vi "Alarms Test Bench.vi"() -> ()   [LabVIEW 2014]
uses:
  Controls/Alarms Data.ctl
  Controls/Modbus Status Interface Data MOD2.ctl
panel:
  in  "Clear Alarms In":bool=TRUE
  in  "MSI Data":T1 {"Converter Faults (30056)" format="%016b"; "Solar Faults (30057)" format="%016b"; "ES Rack 10 Alarms (30120)" format="%016b"; "ES Rack 9 Alarms (30119)" format="%016b"; "ES Rack 8 Alarms (30118)" format="%016b"; "ES Rack 7 Alarms (30117)" format="%016b"; "ES Rack 6 Alarms (30116)" format="%016b"; "ES Rack 5 Alarms (30115)" format="%016b"; "ES Rack 4 Alarms (30114)" format="%016b"; "ES Rack 3 Alarms (30113)" format="%016b"; "ES Rack 2 Alarms (30112)" format="%016b"; "ES Rack 1 Alarms (30111)" format="%016b"; "ES System Alarms (30055)" format="%016b"; "System Faults (30052)" format="%016b"; "ES Rack 10 Faults (30110)" format="%016b"; "Es Rack 9 Faults (30109)" format="%016b"; "ES Rack 8 Faults (30108)" format="%016b"; "ES Rack 7  Faults (30107)" format="%016b"; "ES Rack 6 Faults (30106)" format="%016b"; "ES Rack 5 Faults (30105)" format="%016b"; "ES Rack 4 Faults (30104)" format="%016b"; "ES Rack 3 Faults (30103)" format="%016b"; "ES Rack 2 Faults (30102)" format="%016b"; "ES Rack 1 Faults (30101)" format="%016b"; "ES System Faults (30054)" format="%016b"; "System Status (30051)" format="%016b"; "Controller Faults (30053)" format="%016b"}
  out "Alarms Data Out":T2
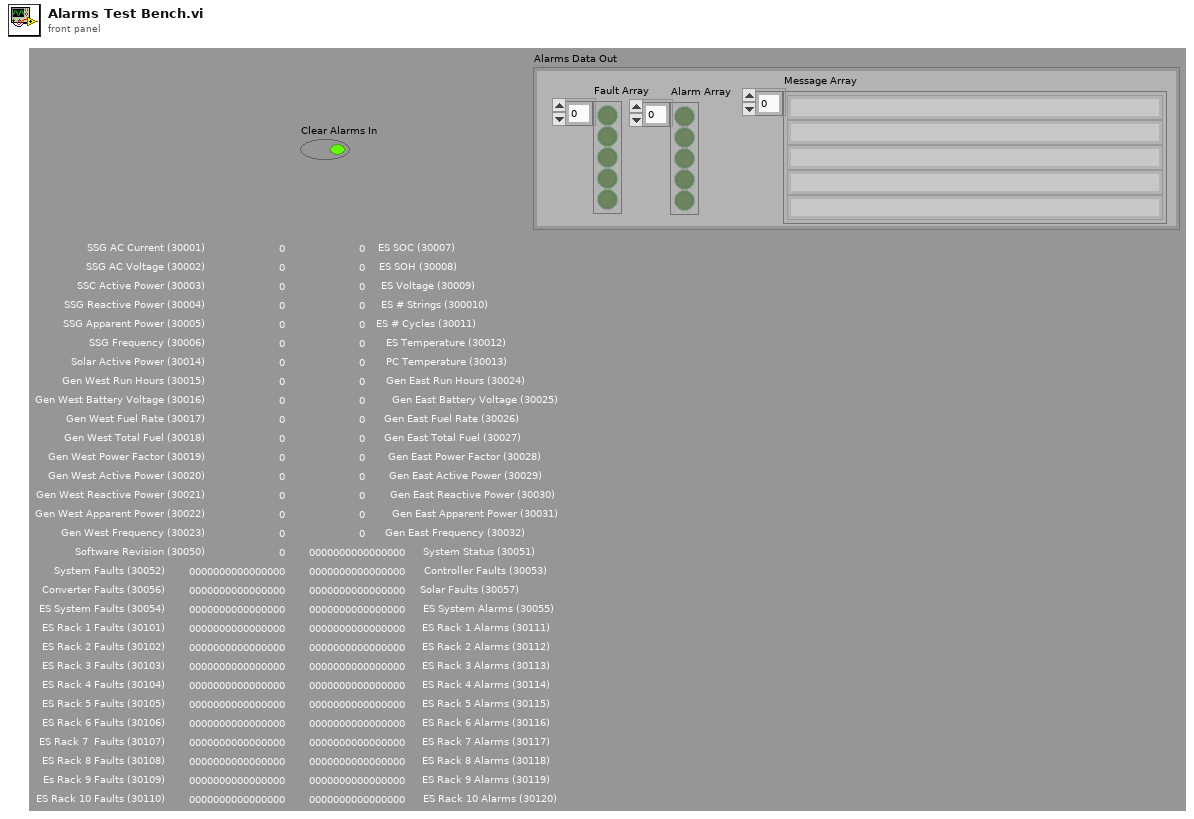
[diagram p1: front panel]
types:
  T1 = typedef "Modbus Status Interface Data MOD2.ctl" = cluster{"SSG AC Current (30001)":i16, "SSG AC Voltage (30002)":i16, "SSC Active Power (30003)":i16, "SSG Reactive Power (30004)":i16, "SSG Apparent Power (30005)":i16, "SSG Frequency (30006)":i16, "ES SOC (30007)":i16, "ES SOH (30008)":i16, "ES Voltage (30009)":i16, "ES # Strings (300010)":i16, "ES # Cycles (30011)":i16, "ES Temperature (30012)":i16, "PC Temperature (30013)":i16, "Solar Active Power (30014)":i16, "Gen West Run Hours (30015)":i16, "Gen West Battery Voltage (30016)":i16, "Gen West Fuel Rate (30017)":i16, "Gen West Total Fuel (30018)":i16, "Gen West Power Factor (30019)":i16, "Gen West Active Power (30020)":i16, "Gen West Reactive Power (30021)":i16, "Gen West Apparent Power (30022)":i16, "Gen West Frequency (30023)":i16, "Gen East Run Hours (30024)":i16, "Gen East Battery Voltage (30025) ":i16, "Gen East Fuel Rate (30026)":i16, "Gen East Total Fuel (30027)":i16, "Gen East Power Factor (30028)":i16, "Gen East Active Power (30029)":i16, "Gen East Reactive Power (30030)":i16, "Gen East Apparent Power (30031)":i16, "Gen East Frequency (30032)":i16, "Software Revision (30050)":i16, "Controller Faults (30053)":i16, "System Status (30051)":i16, "ES System Faults (30054)":i16, "ES Rack 1 Faults (30101)":i16, "ES Rack 2 Faults (30102)":i16, "ES Rack 3 Faults (30103)":i16, "ES Rack 4 Faults (30104)":i16, "ES Rack 5 Faults (30105)":i16, "ES Rack 6 Faults (30106)":i16, "ES Rack 7  Faults (30107)":i16, "ES Rack 8 Faults (30108)":i16, "Es Rack 9 Faults (30109)":i16, "ES Rack 10 Faults (30110)":i16, "System Faults (30052)":i16, "ES System Alarms (30055)":i16, "ES Rack 1 Alarms (30111)":i16, "ES Rack 2 Alarms (30112)":i16, "ES Rack 3 Alarms (30113)":i16, "ES Rack 4 Alarms (30114)":i16, "ES Rack 5 Alarms (30115)":i16, "ES Rack 6 Alarms (30116)":i16, "ES Rack 7 Alarms (30117)":i16, "ES Rack 8 Alarms (30118)":i16, "ES Rack 9 Alarms (30119)":i16, "ES Rack 10 Alarms (30120)":i16, "Solar Faults (30057)":i16, "Converter Faults (30056)":i16}
  T2 = typedef "Alarms Data.ctl" = cluster{"Message Array":string[], "Fault Array":bool[], "Alarm Array":bool[]}
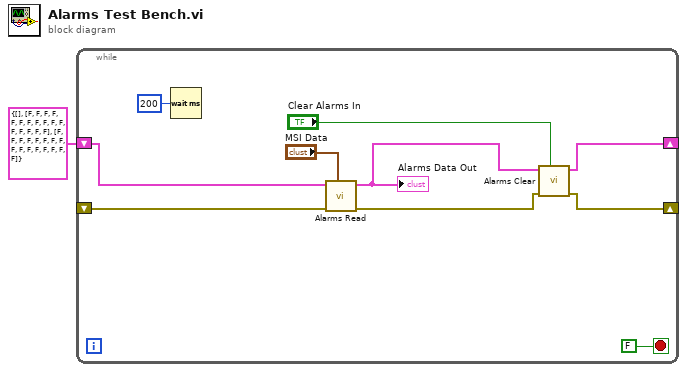
[diagram p0: block diagram]
diagram:
  n1 = while {
    shift-right: [w3] -> _
    shift-left: _ -> [w11]
    shift-right: [w5] -> _
    shift-left: T2 {"Message Array"=[], "Fault Array"=[FALSE, FALSE, FALSE, FALSE, FALSE, FALSE, FALSE, FALSE, FALSE, FALSE, FALSE, FALSE, FALSE, FALSE, FALSE, FALSE], "Alarm Array"=[FALSE, FALSE, FALSE, FALSE, FALSE, FALSE, FALSE, FALSE, FALSE, FALSE, FALSE, FALSE, FALSE, FALSE, FALSE, FALSE]} ("Alarms Data Out") -> [w7]
    stop <- FALSE stop-if-true
    n2 = Wait (ms)(milliseconds to wait=u32 200) -> ()  [unwired: 1 out]
    n3 = call "Alarms Read.vi"("MSI Data"="MSI Data", "Error In"=w11, "Alarms Data In"=w7) -> ("Error Out"=w4:errorcluster, "Alarms Data Out"=w6:T2)  [unwired: 7 in]
    "Alarms Data Out" <- w6
    n4 = call "Alarms Clear.vi"("Clear Alarms In"="Clear Alarms In", "Error In"=w4, "Alarms Data In"=w6) -> ("Error Out"=w3:errorcluster, "Alarms Data Out"=w5:T2)  [unwired: 7 in]
  }
